vi "Write Excluded Tests.vi"(8 "error in (no error)":errorcluster, 10 "Excluded Tests":path[](array[path]), 11 "Test Runner in":refnum<class "Test Runner.lvclass">) -> (0 "error out":errorcluster, 3 "Test Runner out":refnum<class "Test Runner.lvclass">)   [LabVIEW 2020, in "Caraya.lvlib" / "Test Runner.lvclass"]
uses:
  Test Runner.lvclass
  Test Runner.lvclass/Test Runner.ctl
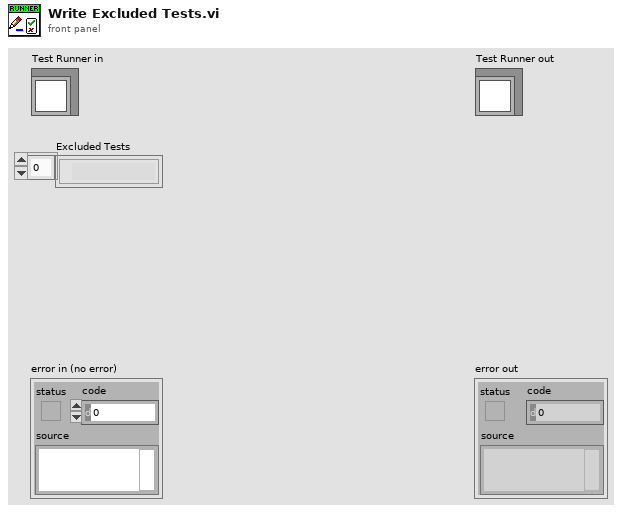
[diagram p1: front panel]
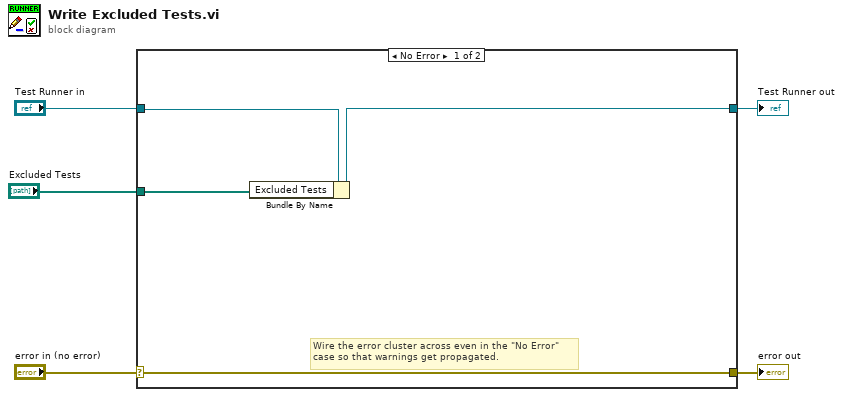
[diagram p0: block diagram]
diagram:
  n1 = case shown="No Error" "error in (no error)" {
    selector: "error in (no error)" -> [w9 w11]
    tunnel: [w9 w11] -> w4
    tunnel: [w6 w10] -> w2
    tunnel: "Test Runner in" -> [w8 w10]
    tunnel: "Excluded Tests" -> [w7 _]
    frame No Error {
      # "Wire the error cluster across even in the \"No Error\"\ncase so that warnings get propagated."
      n2 = Bundle By Name(cluster=w8, "Excluded Tests"=w7) -> (w6:refnum<class "Test Runner.lvclass">)
    }
    frame Error {
    }
  }
  "error out" <- w4
  "Test Runner out" <- w2
